vi "WFM MNGR Create ET Waveform.vi"(0 "WFM MNGR in":refnum<class "QPA MSMT Waveform Manager.lvclass">, 5 "RF Waveform Alias":string, 7 "Vmin":dbl, 9 "Vmax":dbl, 11 "error in (no error)":errorcluster) -> (4 "WFM MNGR out":refnum<class "QPA MSMT Waveform Manager.lvclass">, 6 "ET Waveform":T1, 15 "error out":errorcluster)   [LabVIEW 2016, in "QPA MSMT Waveform Manager.lvclass"]
uses:
  QPA MSMT Waveform Manager.lvclass
  Controls/ET Waveform.ctl
  QPA MSMT Waveform Manager.lvclass/QPA MSMT Waveform Manager.ctl
  Controls/RF Waveform.ctl
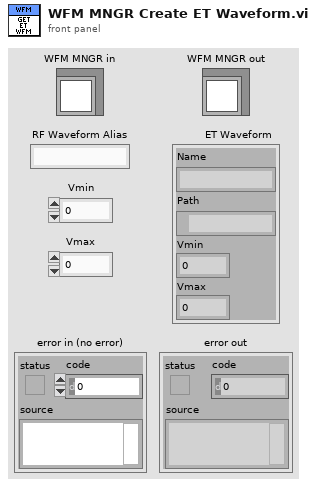
[diagram p1: front panel]
types:
  T1 = typedef "QPA MSMT Waveform Manager.lvclass/ET Waveform.ctl" = cluster{"Name":string, "Path":path, "Vmin":dbl, "Vmax":dbl}
  T2 = typedef "QPA MSMT Waveform Manager.lvclass/RF Waveform.ctl" = cluster{"Name":string, "Path":path, "Headroom":dbl, "Burst Length":dbl}
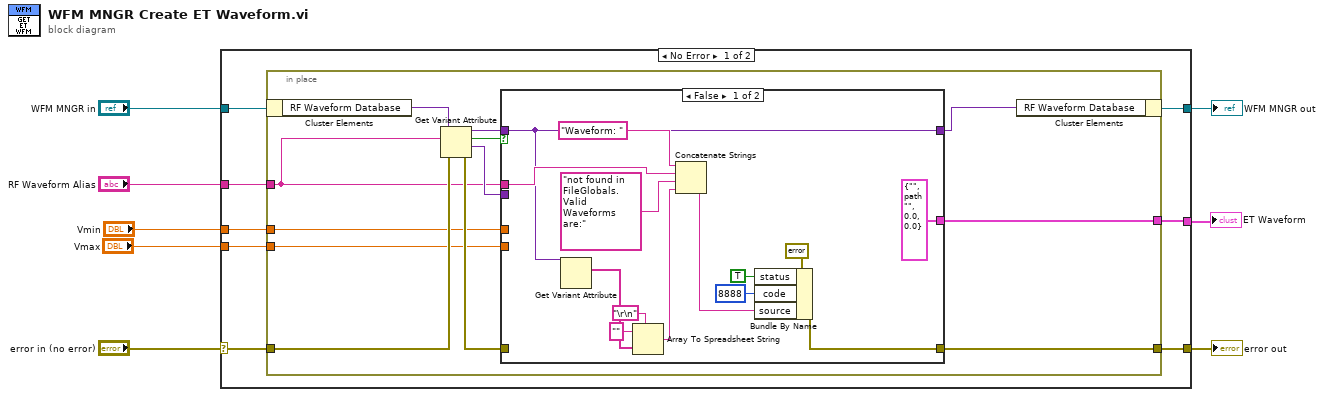
[diagram p0: block diagram]
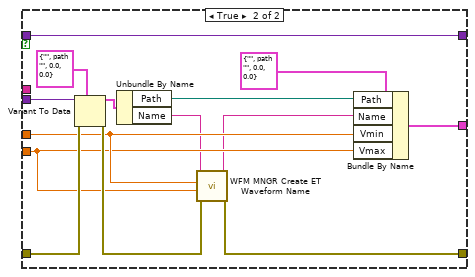
[diagram p2: hidden frame]
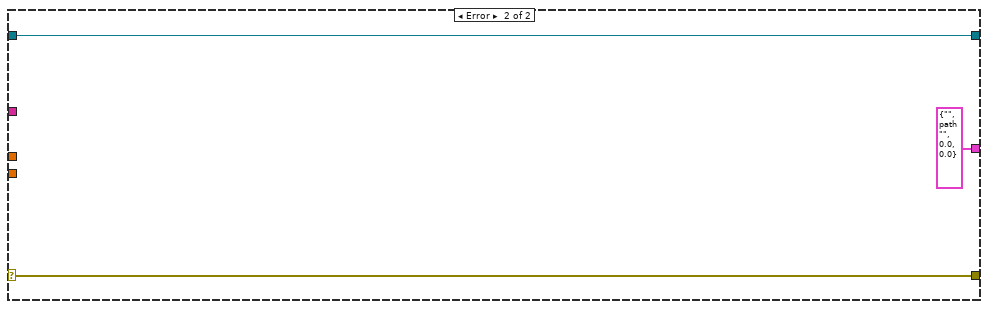
[diagram p3: hidden frame]
diagram:
  n1 = case shown="No Error" "error in (no error)" {
    selector: "error in (no error)" -> [w14 w59]
    tunnel: [w13 w59] -> w7
    tunnel: [w15 w58] -> w5
    tunnel: "WFM MNGR in" -> [w16 w58]
    tunnel: "RF Waveform Alias" -> [w12 _]
    tunnel: [w9 T1 {"Name"="", "Path"=path "", "Vmin"=0.0, "Vmax"=0.0} ("ET Waveform")] -> w1
    tunnel: "Vmin" -> [w11 _]
    tunnel: "Vmax" -> [w10 _]
    frame No Error {
      n2 = in-place {
        in-place-border: w14 -> [w27]
        in-place-border: [w18] -> w13
        in-place-border: w12 -> [w23]
        in-place-border: w11 -> [w20]
        in-place-border: w10 -> [w19]
        in-place-border: [w17] -> w9
        n3 = in-place-cluster #1(w16) -> ("RF Waveform Database"=w28:variant)
        n4 = Get Variant Attribute(Variant=w28, name=w23, error in=w27) -> (duplicate Variant=w22:variant, found=w24:bool, value=w26:variant, error out=w25:errorcluster)  [unwired: 1 in]
        n5 = case shown="False" w24 {
          tunnel: w26 -> [_ w56]
          tunnel: w25 -> [_ w55]
          tunnel: [w31 w50] -> w18
          tunnel: w23 -> [w32 _]
          tunnel: w22 -> [w30 w53]
          tunnel: [w30 w53] -> w21
          tunnel: w20 -> [_ w48]
          tunnel: w19 -> [_ w47]
          tunnel: [T1 {"Name"="", "Path"=path "", "Vmin"=0.0, "Vmax"=0.0} ("ET Waveform") w43] -> w17
          frame False {
            n6 = Get Variant Attribute(Variant=w30) -> (names=w37:string[])  [unwired: 3 in, 3 out]
            n7 = Array To Spreadsheet String(delimiter (Tab)="\r\n", array=w37, 3:"" ("format string")) -> (spreadsheet string=w35:string)
            n8 = Concatenate Strings("Waveform: " ("source"), w32, "not found in FileGlobals.  Valid Waveforms are:" ("string"), w35) -> (w34:string)
            n9 = Bundle By Name(cluster=errorcluster {"status"=FALSE, "code"=0, "source"=""} ("error out"), "status"=TRUE, "code"=8888, "source"=w34) -> (w31:errorcluster)
          }
          frame True {
            n10 = Variant To Data(error in=w55, type=T2 {"Name"="", "Path"=path "", "Headroom"=0.0, "Burst Length"=0.0} ("RF Waveform"), Variant=w56) -> (data=w52:T2, error out=w51:errorcluster)
            n11 = Unbundle By Name(w52) -> ("Path"=w46:path, "Name"=w45:string)
            n12 = call "WFM MNGR Create ET Waveform Name.vi"("error in (no error)"=w51, "Vmax"=w47, "Vmin"=w48, "Name"=w45) -> ("error out"=w50:errorcluster, "result string"=w44:string)  [unwired: 4 in]
            n13 = Bundle By Name(cluster=T1 {"Name"="", "Path"=path "", "Vmin"=0.0, "Vmax"=0.0} ("ET Waveform"), "Path"=w46, "Name"=w44, "Vmin"=w48, "Vmax"=w47) -> (w43:T1)
          }
        }
        n14 = in-place-cluster #1("RF Waveform Database"=w21) -> (w15:refnum<class "QPA MSMT Waveform Manager.lvclass">)
      }
    }
    frame Error {
    }
  }
  "error out" <- w7
  "WFM MNGR out" <- w5
  "ET Waveform" <- w1
